vi "XML_EEG_readDocumentRef.vi"(8 "error in (no error)":errorcluster, 11 "XML_EEG_File in":refnum<class "XML_EEG_File.lvclass">) -> (0 "error out":errorcluster, 2 "DOM document Ref":refnum<k20>, 3 "XML_EEG_File out":refnum<class "XML_EEG_File.lvclass">)   [LabVIEW 2016, in "XML_EEG_File_Parser.lvlib" / "XML_EEG_File.lvclass"]
uses:
  XML_EEG_File.lvclass
  XML_EEG_File.lvclass/XML_EEG_File.ctl
panel:
  # "This VI is a part of BCI Design library, http://www.ru-bci.org \nCopyright © 2020, Sotnikov Peter, All rights reserved. License: GNU GPLv3"
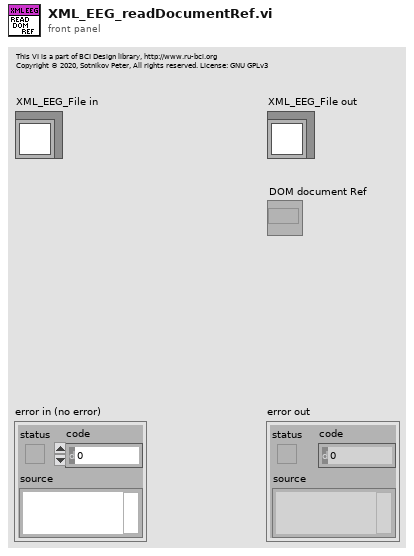
[diagram p1: front panel]
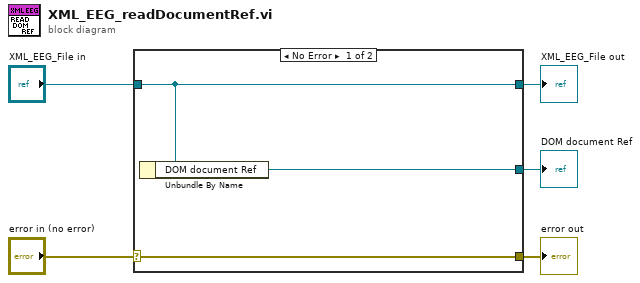
[diagram p0: block diagram]
diagram:
  n1 = case shown="No Error" "error in (no error)" {
    selector: "error in (no error)" -> [w8 w9]
    tunnel: [w8 w9] -> w4
    tunnel: [w7 w10] -> w2
    tunnel: "XML_EEG_File in" -> [w7 w10]
    tunnel: [w6 _] -> w1
    frame No Error {
      n2 = Unbundle By Name(w7) -> ("DOM document Ref"=w6:refnum<k20>)
    }
    frame Error {
    }
  }
  "error out" <- w4
  "XML_EEG_File out" <- w2
  "DOM document Ref" <- w1
